vi "Large integer U8 array - divide by 2.vi"(5 "Large number - U8":T1) -> (1 "Divided by 2":T1)   [LabVIEW 2012]
doc: "Rotates down 1 bit all bits in a large numbers (U8 array format)."
uses:
  User Access Type defs/Large number - U8 array.ctl
panel:
  # "index 0 = LSD"
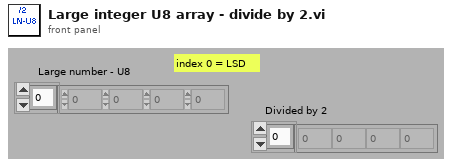
[diagram p1: front panel]
types:
  T1 = typedef "Large number - U8 array.ctl" = u8[]
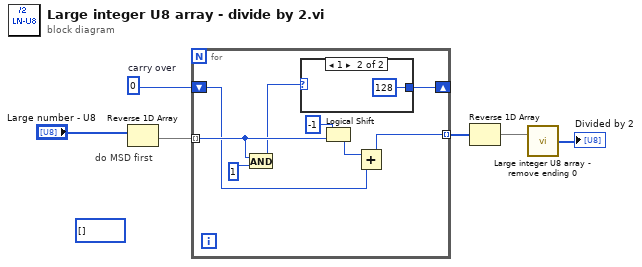
[diagram p0: block diagram]
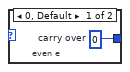
[diagram p2: hidden frame]
diagram:
  w6 = u8 0  # carry over
  (unwired) T1 [] ("Added array")
  # "do MSD first"
  n1 = Reverse 1D Array(array="Large number - U8") -> (reversed array=w4:T1)
  n2 = for {
    shift-right: [w10] -> _
    shift-left: w6 -> [w8]
    tunnel: w4 -> [w12] mode=indexing
    tunnel: [w7] -> w3 mode=indexing
    n3 = And(x=w12, y=u32 1) -> (x .and. y?=w11:u32)
    n4 = case shown="1" w11 {
      tunnel: [w15 u8 128 ("carry over")] -> w10
      frame 0, Default {
        w15 = u8 0  # carry over
        # "even e"
      }
      frame 1 {
      }
    }
    n5 = Logical Shift(y=-1, x=w12) -> (x << y=w9:u8)
    n6 = Add(x=w9, y=w8) -> (x+y=w7:u8)
  }
  n7 = Reverse 1D Array(array=w3) -> (reversed array=w2:u8[])
  n8 = call "Large integer U8 array - remove ending 0.vi"("Large number - U8"=w2) -> ("MSD zeros removed"=→"Divided by 2":T1)  [unwired: 4 out]
